vi "Sequence jsObject.vi"(8 "error in (no error)":errorcluster, 9 "Sequence Record (empty)":T1, 10 "Sequence jsObject Name (\"\")":string, 11 "Previous String (\"\")":string) -> (0 "error out":errorcluster, 2 "Sequence jsObject":string, 3 "SEQUENCE jsObject Definition":string)   [LabVIEW 2011]
uses:
  Sequence Record.ctl
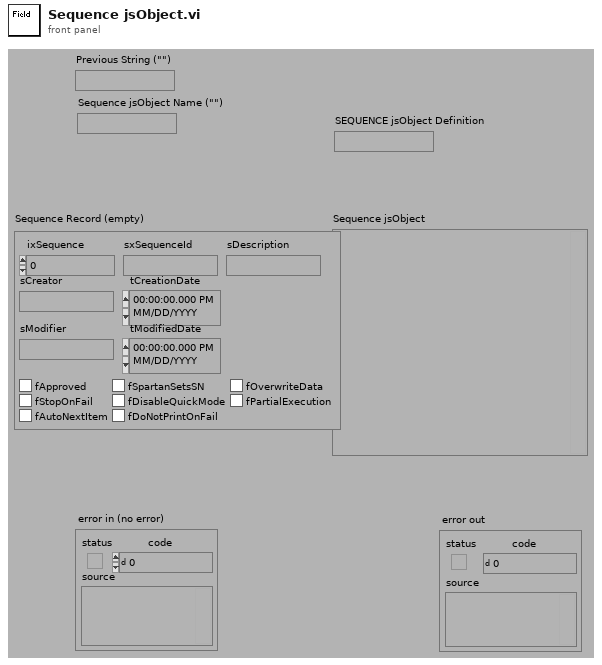
[diagram p1: front panel]
types:
  T1 = typedef "Sequence Record.ctl" = cluster{"ixSequence":i32, "sxSequenceId":string, "sDescription":string, "sCreator":string, "tCreationDate":timestamp, "sModifier":string, "tModifiedDate":timestamp, "fApproved":bool, "fSpartanSetsSN":bool, "fOverwriteData":bool, "fStopOnFail":bool, "fDisableQuickMode":bool, "fPartialExecution":bool, "fAutoNextItem":bool, "fDoNotPrintOnFail":bool}
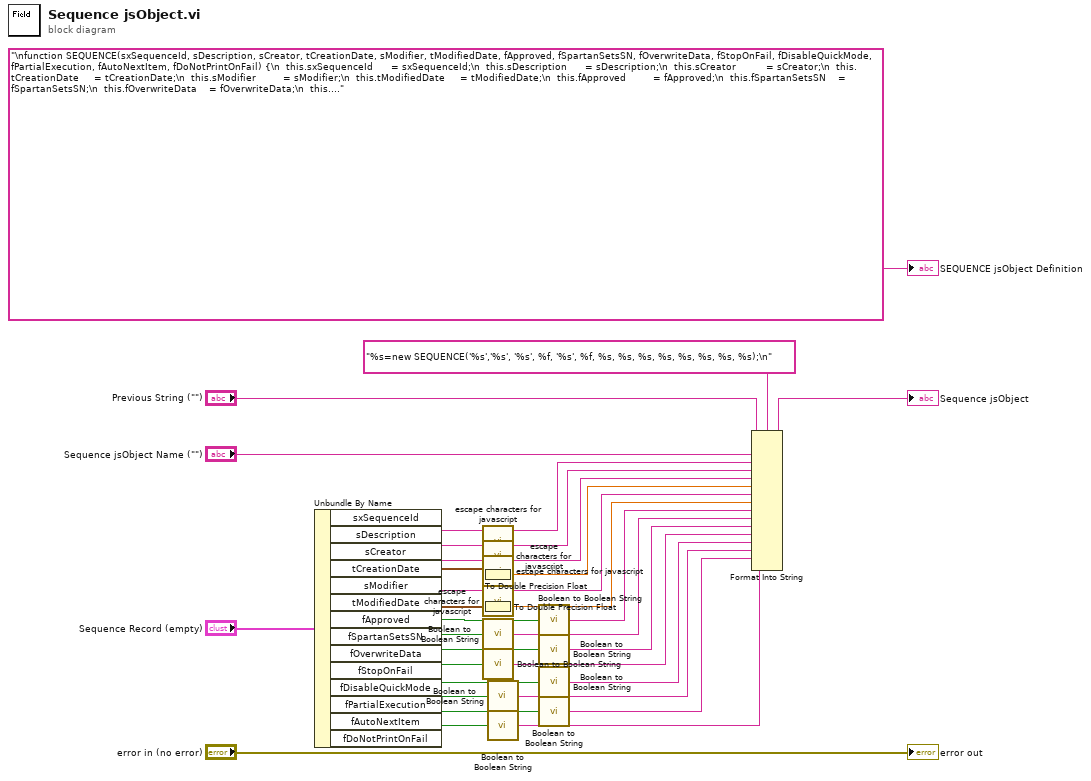
[diagram p0: block diagram]
diagram:
  n1 = Unbundle By Name("Sequence Record (empty)") -> ("sxSequenceId"=w31:string, "sDescription"=w29:string, "sCreator"=w27:string, "tCreationDate"=w25:timestamp, "sModifier"=w23:string, "tModifiedDate"=w21:timestamp, "fApproved"=w17:bool, "fSpartanSetsSN"=w15:bool, "fOverwriteData"=w14:bool, "fStopOnFail"=w13:bool, "fDisableQuickMode"=w12:bool, "fPartialExecution"=w11:bool, "fAutoNextItem"=w10:bool, "fDoNotPrintOnFail"=w2:bool)
  n2 = call "escape characters for javascript.vi"("String (\"\")"=w31) -> ("escaped String"=w30:string)  [unwired: 4 out]
  n3 = call "escape characters for javascript.vi"("String (\"\")"=w29) -> ("escaped String"=w28:string)  [unwired: 4 out]
  n4 = call "escape characters for javascript.vi"("String (\"\")"=w27) -> ("escaped String"=w26:string)  [unwired: 4 out]
  n5 = To Double Precision Float(number=w25) -> (double precision float=w24:dbl)
  n6 = call "escape characters for javascript.vi"("String (\"\")"=w23) -> ("escaped String"=w22:string)  [unwired: 4 out]
  n7 = To Double Precision Float(number=w21) -> (double precision float=w20:dbl)
  n8 = call "Boolean to Boolean String.vi"("Boolean"=w15) -> ("Boolean string"=w9:string)  [unwired: 1 in]
  n9 = call "Boolean to Boolean String.vi"("Boolean"=w13) -> ("Boolean string"=w7:string)  [unwired: 1 in]
  n10 = call "Boolean to Boolean String.vi"("Boolean"=w11) -> ("Boolean string"=w5:string)  [unwired: 1 in]
  n11 = call "Boolean to Boolean String.vi"("Boolean"=w2) -> ("Boolean string"=w1:string)  [unwired: 1 in]
  n12 = call "Boolean to Boolean String.vi"("Boolean"=w17) -> ("Boolean string"=w16:string)  [unwired: 1 in]
  n13 = call "Boolean to Boolean String.vi"("Boolean"=w14) -> ("Boolean string"=w8:string)  [unwired: 1 in]
  n14 = call "Boolean to Boolean String.vi"("Boolean"=w12) -> ("Boolean string"=w6:string)  [unwired: 1 in]
  n15 = call "Boolean to Boolean String.vi"("Boolean"=w10) -> ("Boolean string"=w4:string)  [unwired: 1 in]
  n16 = Format Into String(format string="%s=new SEQUENCE('%s','%s', '%s', %f, '%s', %f, %s, %s, %s, %s, %s, %s, %s, %s);\n", initial string="Previous String (\"\")", "Sequence jsObject Name (\"\")", w30, w28, w26, w24, w22, w20, w16, w9, w8, w7, w6, w5, w4, w1) -> (resulting string=→"Sequence jsObject":string)  [unwired: 1 in, 1 out]
  "error out" <- "error in (no error)"
  "SEQUENCE jsObject Definition" <- "\nfunction SEQUENCE(sxSequenceId, sDescription, sCreator, tCreationDate, sModifier, tModifiedDate, fApproved, fSpartanSetsSN, fOverwriteData, fStopOnFail, fDisableQuickMode, fPartialExecution, fAutoNextItem, fDoNotPrintOnFail) {\n  this.sxSequenceId      = sxSequenceId;\n  this.sDescription      = sDescription;\n  this.sCreator          = sCreator;\n  this.tCreationDate     = tCreationDate;\n  this.sModifier         = sModifier;\n  this.tModifiedDate     = tModifiedDate;\n  this.fApproved         = fApproved;\n  this.fSpartanSetsSN    = fSpartanSetsSN;\n  this.fOverwriteData    = fOverwriteData;\n  this.fStopOnFail       = fStopOnFail;  \n  this.fDisableQuickMode = fDisableQuickMode; \n  this.fPartialExecution = fPartialExecution;  \n  this.fAutoNextItem     = fAutoNextItem;\n  this.fDoNotPrintOnFail = fDoNotPrintOnFail;\n}\n"
